vi "Array2DtoTwoArrays1D.vi"(4 "Input (2D array)":dbl[][](array[numeric])) -> (0 "Y Data Array":dbl[](array[numeric]), 1 "X Data Array":dbl[](array[numeric]))   [LabVIEW 2017]
doc: "Takes a 2 D array and generates 2 1D arrays."
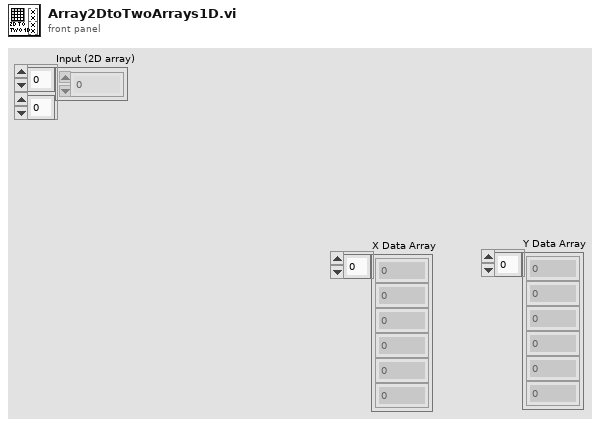
[diagram p1: front panel]
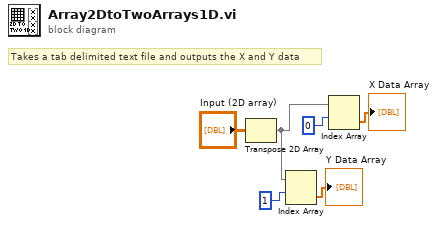
[diagram p0: block diagram]
diagram:
  # "Takes a tab delimited text file and outputs the X and Y data"
  n1 = Transpose 2D Array(2D array="Input (2D array)") -> (transposed array=w3:dbl[][])
  n2 = Index Array(array=w3, index (row)=1 ("indexX")) -> (element=→"Y Data Array":dbl[])  [unwired: 1 in]
  n3 = Index Array(array=w3, index (row)=0 ("indexX")) -> (element=→"X Data Array":dbl[])  [unwired: 1 in]
